vi "testAppendCircArr.vi"(8 "error in (no error)":errorcluster) -> (0 "error out":errorcluster)   [LabVIEW 2016]
doc: "Test to append the circular array."
uses:
  MatOper/appendCircStrArr.vi
  MatOper/appendCircNumArr.vi
  <vilib>/addons/_JKI Toolkits/Caraya/classes/Test/Test.lvclass
  MatOper/MatOper.lvclass
  <vilib>/addons/_JKI Toolkits/Caraya/classes/Assert/Assert.lvclass
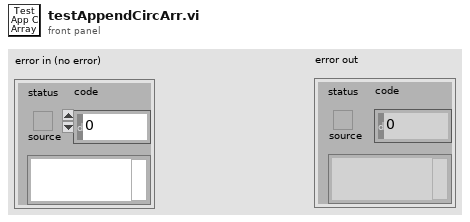
[diagram p1: front panel]
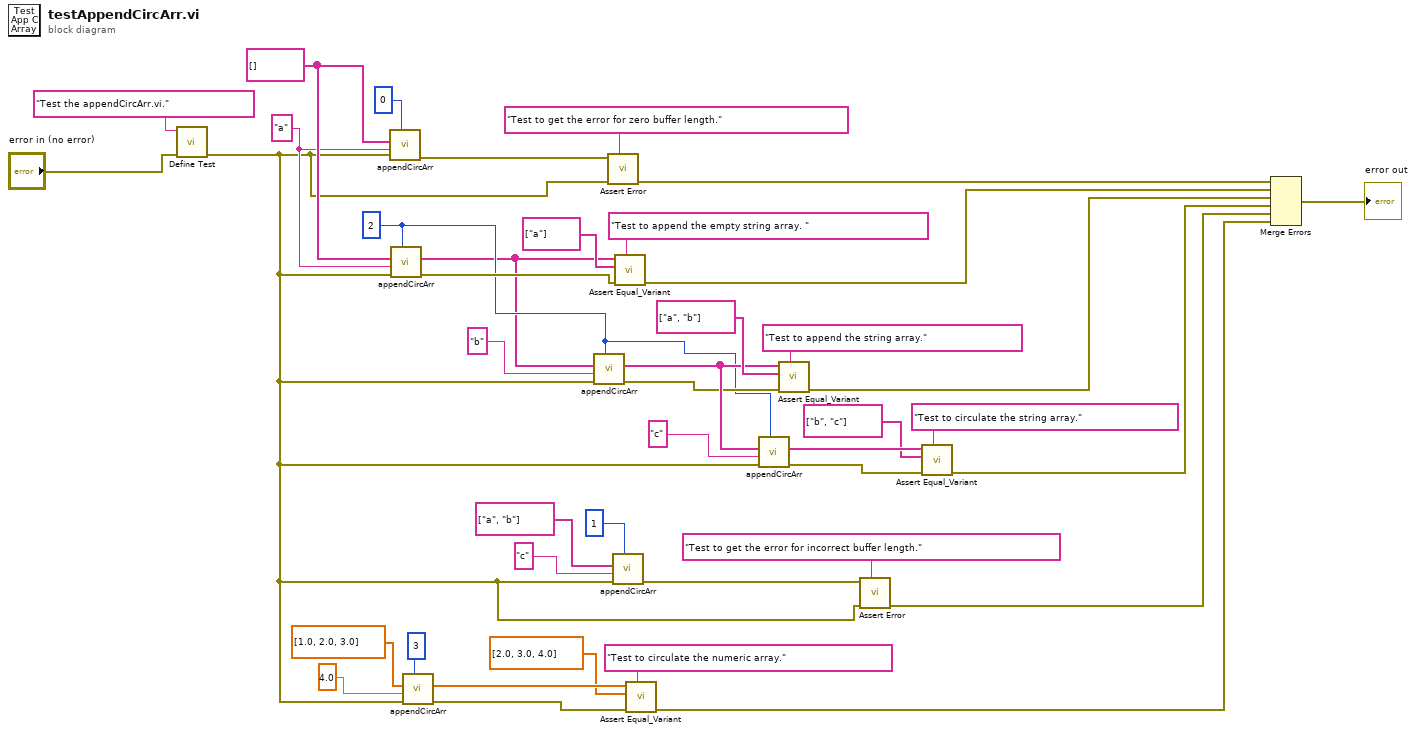
[diagram p0: block diagram]
diagram:
  w23 = 2
  w36 = "a"
  w37 = string[] []
  n1 = call <vilib>:"Define Test.vi"("error in (no error)"="error in (no error)", "Label (VI Title)"="Test the appendCircArr.vi.") -> ("error out"=w4:errorcluster)  [unwired: 9 in]
  n2 = call-poly "appendCircArr.vi"("Buffer Length"=0, "error in (no error)"=w4, "New String"=w36, "String Array"=w37) -> ("error out"=w38:errorcluster)  [unwired: 5 in, 2 out]
  n3 = call-poly "appendCircArr.vi"("Buffer Length"=w23, "error in (no error)"=w4, "New String"=w36, "String Array"=w37) -> ("error out"=w34:errorcluster, "Updated String Array"=w10:string[])  [unwired: 5 in, 1 out]
  n4 = call-poly "appendCircArr.vi"("Buffer Length"=3, "error in (no error)"=w4, "New Numeric"=4.0, "Numeric Array"=dbl[] [1.0, 2.0, 3.0]) -> ("error out"=w13:errorcluster, "Updated Numeric Array"=w14:dbl[])  [unwired: 5 in, 1 out]
  n5 = call-poly "appendCircArr.vi"("Buffer Length"=w23, "error in (no error)"=w4, "New String"="b", "String Array"=w10) -> ("error out"=w25:errorcluster, "Updated String Array"=w26:string[])  [unwired: 5 in, 1 out]
  n6 = call <vilib>:"Assert Error.vi"("Label"="Test to get the error for zero buffer length.", "error in (no error)"=w4, "Error?"=w38) -> ("error out"=w32:errorcluster)  [unwired: 8 in]
  n7 = call-poly "appendCircArr.vi"("Buffer Length"=1, "error in (no error)"=w4, "New String"="c", "String Array"=string[] ["a", "b"]) -> ("error out"=w5:errorcluster)  [unwired: 5 in, 2 out]
  n8 = call <vilib>:"Assert Equal_Variant.vi"("Label"="Test to append the empty string array. ", "error in (no error)"=w34, "Y"=string[] ["a"], "X"=w10) -> ("error out"=w31:errorcluster)  [unwired: 7 in]
  n9 = call <vilib>:"Assert Equal_Variant.vi"("Label"="Test to circulate the numeric array.", "error in (no error)"=w13, "Y"=dbl[] [2.0, 3.0, 4.0], "X"=w14) -> ("error out"=w1:errorcluster)  [unwired: 7 in]
  n10 = call-poly "appendCircArr.vi"("Buffer Length"=w23, "error in (no error)"=w4, "New String"="c", "String Array"=w26) -> ("error out"=w21:errorcluster, "Updated String Array"=w22:string[])  [unwired: 5 in, 1 out]
  n11 = call <vilib>:"Assert Equal_Variant.vi"("Label"="Test to append the string array.", "error in (no error)"=w25, "Y"=string[] ["a", "b"], "X"=w26) -> ("error out"=w29:errorcluster)  [unwired: 7 in]
  n12 = call <vilib>:"Assert Error.vi"("Label"="Test to get the error for incorrect buffer length.", "error in (no error)"=w4, "Error?"=w5) -> ("error out"=w2:errorcluster)  [unwired: 8 in]
  n13 = call <vilib>:"Assert Equal_Variant.vi"("Label"="Test to circulate the string array.", "error in (no error)"=w21, "Y"=string[] ["b", "c"], "X"=w22) -> ("error out"=w19:errorcluster)  [unwired: 7 in]
  n14 = Merge Errors(w32, w31, w29, w19, w2, w1) -> (→"error out":errorcluster)
